vi "Poll for Fault Code Condition.vi"(0 "GEA2 Reference In":refnum<k24>, 5 "Fault ID (Decimal)":u16, 7 "Fault Status (00/FF)":string="00", 9 "Query Rate (ms)":u32=5, 11 "Error In":errorcluster, 12 "Timeout (s)":dbl) -> (4 "GEA2 Reference Out":refnum<k24>, 6 "Pass/Fail?":bool, 8 "Report Text":string, 10 "Time to fault code set (s)":dbl, 15 "Error Out":errorcluster)   [LabVIEW 2016, in "TLMB.lvlib"]
uses:
  Projects/TLMB.lvlib
  Q:/Common/DLLs/GEA3/GeaCommunication.dll
  Common/DLLs/GEA3/GeaCommunication.dll
  Common/LabVIEW GEA2 Toolkit/LabVIEW_GEA2_Toolkit.lvlibp/type defs/Source_Destination.ctl
  Common/LabVIEW GEA2 Toolkit/LabVIEW_GEA2_Toolkit.lvlibp
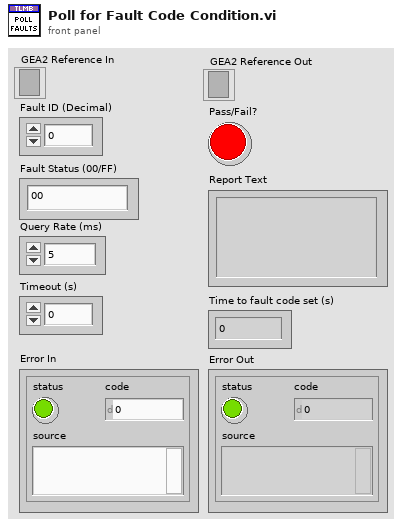
[diagram p1: front panel]
types:
  T1 = typedef "LabVIEW_GEA2_Toolkit.lvlibp/Source_Destination.ctl" = cluster{"Source":u8, "Destination":u8}
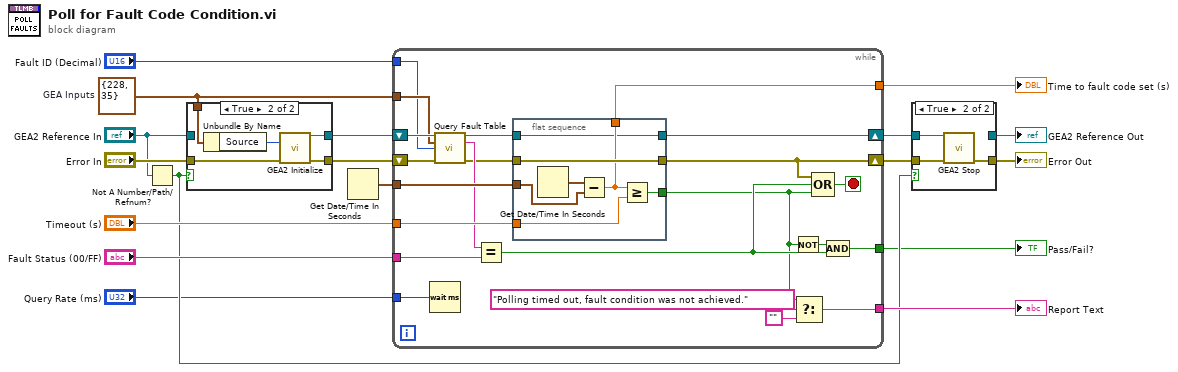
[diagram p0: block diagram]
diagram:
  w13 = T1 {"Source"=228, "Destination"=35}  # GEA Inputs
  n1 = Not A Number/Path/Refnum?(number/path/refnum="GEA2 Reference In") -> (NaN/Path/Refnum?=w4:bool)
  n2 = case shown="True" w4 {
    tunnel: w13 -> [_ w25]
    tunnel: "Error In" -> [w20 w23]
    tunnel: [w20 w22] -> w11
    tunnel: [w19 w21] -> w10
    tunnel: "GEA2 Reference In" -> [w19 _]
    frame False {
    }
    frame True {
      n3 = Unbundle By Name(w25) -> ("Source"=w24:u8)
      n4 = call "GEA2 Initialize.vi"("Source Address"=w24, "error in"=w23) -> ("GEA2 Reference Out"=w21:refnum<k24>, "error out"=w22:errorcluster)  [unwired: 11 in, 1 out]
    }
  }
  n5 = Get Date/Time In Seconds() -> (seconds since 1Jan1904=w17:timestamp)
  n6 = while {
    tunnel: "Fault Status (00/FF)" -> [w47]
    tunnel: w13 -> [w38]
    shift-right: [w36] -> w5
    shift-left: w11 -> [w39]
    shift-right: [w33] -> w6
    shift-left: w10 -> [w40]
    tunnel: w17 -> [w46]
    tunnel: "Timeout (s)" -> [w45]
    tunnel: [w26] -> w3
    tunnel: [w41] -> w15
    tunnel: [w34] -> w14
    tunnel: "Fault ID (Decimal)" -> [w31]
    tunnel: "Query Rate (ms)" -> [w30]
    stop <- w44 stop-if-true
    n7 = Wait (ms)(milliseconds to wait=w30) -> ()  [unwired: 1 out]
    n8 = call "Query Fault Table.vi"("GEA2 Reference In"=w40, "GEA Inputs"=w38, "Fault ID"=w31, "Error In"=w39) -> ("GEA2 Reference Out"=w32:refnum<k24>, "Fault Status"=w37:string, "Error Out"=w35:errorcluster)  [unwired: 9 in]
    n9 = Equal?(x=w37, y=w47) -> (x = y?=w29:bool)
    n10 = flat-sequence {
      tunnel: w46 -> [w53]
      tunnel: w45 -> [w52]
      tunnel: [w51] -> w28
      tunnel: [w50] -> w36
      tunnel: w35 -> [w50]
      tunnel: [w49] -> w34
      tunnel: [w48] -> w33
      tunnel: w32 -> [w48]
      frame #0 {
        n11 = Get Date/Time In Seconds() -> (seconds since 1Jan1904=w54:timestamp)
        n12 = Subtract(x=w54, y=w53) -> (x-y=w49:dbl)
        n13 = Greater Or Equal?(x=w49, y=w52) -> (x >= y?=w51:bool)
      }
    }
    n14 = Not(x=w28) -> (.not. x?=w27:bool)
    n15 = Select(t="Polling timed out, fault condition was not achieved." ("Fault Code / Set"), s=w28, f="") -> (s? t:f=w41:string)
    n16 = Compound Arithmetic op=OR(w36, w29, w28) -> (w44:bool)
    n17 = Compound Arithmetic op=AND(w27, w29) -> (w26:bool)
  }
  "Report Text" <- w15
  "Time to fault code set (s)" <- w14
  "Pass/Fail?" <- w3
  n18 = case shown="True" w4 {
    tunnel: w5 -> [w56 w59]
    tunnel: [w56 w58] -> w8
    tunnel: [w55 _] -> w7
    tunnel: w6 -> [w55 w57]
    frame False {
    }
    frame True {
      n19 = call "GEA2 Stop.vi"("GEA2 Reference In"=w57, "Error In"=w59) -> ("Error Out"=w58:errorcluster)  [unwired: 13 in]
    }
  }
  "Error Out" <- w8
  "GEA2 Reference Out" <- w7
